vi "subToAbsolutePath.vi"(10 "Path string":string, 11 "Root path":path) -> (3 "Path":path)   [LabVIEW 2019, in "SolutionBuilder.lvlib" / "SolutionBuilder.lvclass"]
uses:
  SolutionBuilder.lvclass
  <vilib>/regexp/Match Regular Expression.xnode
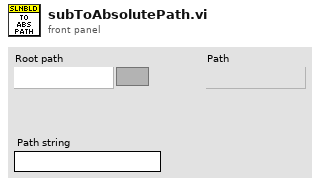
[diagram p1: front panel]
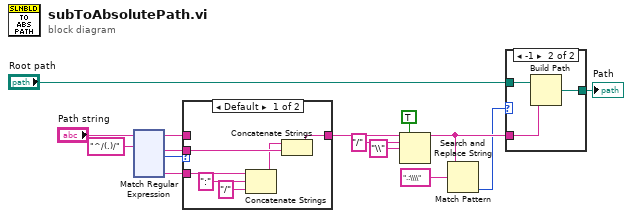
[diagram p0: block diagram]
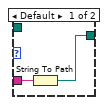
[diagram p3: hidden frame]
diagram:
  n1 = xnode "Match Regular Expression"("input string"="Path string", "regular expression"="^/(.)/") -> ("before match"=w8:string, "after match"=w10:string, "offset past match"=w7:i32, "submatch 1"=w9:string)  [unwired: 4 in, 2 out]
  n2 = case shown="Default" w7 {
    tunnel: w8 -> [_ w22]
    tunnel: [w18 w22] -> w11
    tunnel: w9 -> [w20 _]
    tunnel: w10 -> [w21 _]
    frame Default {
      n3 = Concatenate Strings(w20, ":" ("string"), "/" ("string")) -> (w17:string)
      n4 = Concatenate Strings(w17, w21) -> (w18:string)
    }
    frame -1 {
    }
  }
  n5 = Search and Replace String(replace all?=TRUE ("replace all? (F)"), input string=w11, search string="/", replace string="\\" ("replace string (\"\")")) -> (result string=w12:string)  [unwired: 4 in, 3 out]
  n6 = Match Pattern(string=w12, regular expression=".:\\\\") -> (offset past match=w2:i32)  [unwired: 1 in, 3 out]
  n7 = case shown="-1" w2 {
    tunnel: "Root path" -> [_ w27]
    tunnel: w12 -> [w23 w26]
    tunnel: [w24 w25] -> w4
    frame Default {
      n8 = String To Path(string=w23) -> (path=w24:path)
    }
    frame -1 {
      n9 = Build Path(base path=w27, name or relative path=w26) -> (appended path=w25:path)
    }
  }
  "Path" <- w4
